vi "Weather Parse Test.vi"() -> ()   [LabVIEW 2020, in "CDM-Config.lvlib"] (continued)
,\n                \"instruction\": null,\n                \"response\": \"Avoid\",\n                \"parameters\": {\n                    \"AWIPSidentifier\": [\n                        \"CWFALU\"\n                    ],\n                    \"WMOidentifier\": [\n                        \"FZAK52 PAFC 031300\"\n                    ],\n                    \"NWSheadline\": [\n                        \"GALE WARNING TODAY\"\n                    ],\n                    \"BLOCKCHANNEL\": [\n                        \"EAS\",\n                        \"NWEM\",\n                        \"CMAS\"\n                    ],\n                    \"VTEC\": [\n                        \"/O.NEW.PAFC.GL.W.5654.251203T1400Z-251204T0200Z/\"\n                    ],\n                    \"eventEndingTime\": [\n                        \"2025-12-03T17:00:00-09:00\"\n                    ]\n                },\n                \"scope\": \"Public\",\n                \"code\": \"IPAWSv1.0\",\n                \"language\": \"en-US\",\n                \"web\": \"http://www.weather.gov\",\n                \"eventCode\": {\n                    \"SAME\": [\n                        \"NWS\"\n                    ],\n                    \"NationalWeatherService\": [\n                        \"GLW\"\n                    ]\n                }\n            }\n        },\n        {\n            \"id\": \"https://api.weather.gov/alerts/urn:oid:2.49.0.1.840.0.16ee1729296b80b5948b72c512c8722f6075ae6c.021.1\",\n            \"type\": \"Feature\",\n            \"geometry\": null,\n            \"properties\": {\n                \"@id\": \"https://api.weather.gov/alerts/urn:oid:2.49.0.1.840.0.16ee1729296b80b5948b72c512c8722f6075ae6c.021.1\",\n                \"@type\": \"wx:Alert\",\n                \"id\": \"urn:oid:2.49.0.1.840.0.16ee1729296b80b5948b72c512c8722f6075ae6c.021.1\",\n                \"areaDesc\": \"Seguam to Adak Bering Side out to 15 NM\",\n                \"geocode\": {\n                    \"SAME\": [\n                        \"058780\"\n                    ],\n                    \"UGC\": [\n                        \"PKZ780\"\n                    ]\n                },\n                \"affectedZones\": [\n                    \"https://api.weather.gov/zones/forecast/PKZ780\"\n                ],\n                \"references\": [],\n                \"sent\": \"2025-12-03T04:00:00-09:00\",\n                \"effective\": \"2025-12-03T04:00:00-09:00\",\n                \"onset\": \"2025-12-03T04:00:00-09:00\",\n                \"expires\": \"2025-12-03T17:00:00-09:00\",\n                \"ends\": \"2025-12-04T05:00:00-09:00\",\n                \"status\": \"Actual\",\n                \"messageType\": \"Alert\",\n                \"category\": \"Met\",\n                \"severity\": \"Moderate\",\n                \"certainty\": \"Likely\",\n                \"urgency\": \"Expected\",\n                \"event\": \"Gale Warning\",\n                \"sender\": \"w-nws.webmaster@noaa.gov\",\n                \"senderName\": \"NWS Anchorage AK\",\n                \"headline\": \"Gale Warning issued December 3 at 4:00AM AKST until December 4 at 5:00AM AKST by NWS Anchorage AK\",\n                \"description\": \"Coastal Waters Forecast for Southwest Alaska+Bristol Bay+The\\nAlaska Peninsula Waters and the Aleutian Islands up to 100 nm out.\\n\\nWind forecasts reflect the predominant speed and direction\\nexpected. Sea forecasts represent an average of the highest\\none-third of the combined wind wave and swell height.\\n\\n.TODAY...N wind 40 kt. Seas 27 ft. Rain.\\n.TONIGHT...N wind 35 kt. Seas 22 ft.\\n.THU...NE wind 25 kt diminishing to 15 kt in the afternoon. Seas\\n16 ft.\\n.THU NIGHT...E wind 15 kt. Seas 10 ft.\\n.FRI...Variable wind 10 kt. Seas 7 ft.\\n.SAT...NE wind 25 kt. Seas 8 ft.\\n.SUN...N wind 30 kt. Seas 20 ft.\",\n                \"instruction\": null,\n                \"response\": \"Avoid\",\n                \"parameters\": {\n                    \"AWIPSidentifier\": [\n                        \"CWFALU\"\n                    ],\n                    \"WMOidentifier\": [\n                        \"FZAK52 PAFC 031300\"\n                    ],\n                    \"NWSheadline\": [\n                        \"GALE WARNING THROUGH TONIGHT\"\n                    ],\n                    \"BLOCKCHANNEL\": [\n                        \"EAS\",\n                        \"NWEM\",\n                        \"CMAS\"\n                    ],\n                    \"VTEC\": [\n                        \"/O.NEW.PAFC.GL.W.5656.251203T1300Z-251204T1400Z/\"\n                    ],\n                    \"eventEndingTime\": [\n                        \"2025-12-04T05:00:00-09:00\"\n                    ]\n                },\n                \"scope\": \"Public\",\n                \"code\": \"IPAWSv1.0\",\n                \"language\": \"en-US\",\n                \"web\": \"http://www.weather.gov\",\n                \"eventCode\": {\n                    \"SAME\": [\n                        \"NWS\"\n                    ],\n                    \"NationalWeatherService\": [\n                        \"GLW\"\n                    ]\n                }\n            }\n        },\n        {\n            \"id\": \"https://api.weather.gov/alerts/urn:oid:2.49.0.1.840.0.16ee1729296b80b5948b72c512c8722f6075ae6c.027.1\",\n            \"type\": \"Feature\",\n            \"geometry\": null,\n            \"properties\": {\n                \"@id\": \"https://api.weather.gov/alerts/urn:oid:2.49.0.1.840.0.16ee1729296b80b5948b72c512c8722f6075ae6c.027.1\",\n                \"@type\": \"wx:Alert\",\n                \"id\": \"urn:oid:2.49.0.1.840.0.16ee1729296b80b5948b72c512c8722f6075ae6c.027.1\",\n                \"areaDesc\": \"Kiska to Attu Bering Side\",\n                \"geocode\": {\n                    \"SAME\": [\n                        \"058786\"\n                    ],\n                    \"UGC\": [\n                        \"PKZ786\"\n                    ]\n                },\n                \"affectedZones\": [\n                    \"https://api.weather.gov/zones/forecast/PKZ786\"\n                ],\n                \"references\": [],\n                \"sent\": \"2025-12-03T04:00:00-09:00\",\n                \"effective\": \"2025-12-03T04:00:00-09:00\",\n                \"onset\": \"2025-12-04T05:00:00-09:00\",\n                \"expires\": \"2025-12-03T17:00:00-09:00\",\n                \"ends\": \"2025-12-04T17:00:00-09:00\",\n                \"status\": \"Actual\",\n                \"messageType\": \"Alert\",\n                \"category\": \"Met\",\n                \"severity\": \"Severe\",\n                \"certainty\": \"Observed\",\n                \"urgency\": \"Immediate\",\n                \"event\": \"Storm Warning\",\n                \"sender\": \"w-nws.webmaster@noaa.gov\",\n                \"senderName\": \"NWS Anchorage AK\",\n                \"headline\": \"Storm Warning issued December 3 at 4:00AM AKST until December 4 at 5:00PM AKST by NWS Anchorage AK\",\n                \"description\": \"Coastal Waters Forecast for Southwest Alaska+Bristol Bay+The\\nAlaska Peninsula Waters and the Aleutian Islands up to 100 nm out.\\n\\nWind forecasts reflect the predominant speed and direction\\nexpected. Sea forecasts represent an average of the highest\\none-third of the combined wind wave and swell height.\\n\\n.TODAY...NE wind 25 kt. Seas 20 ft.\\n.TONIGHT...E wind 30 kt becoming SE 40 kt after midnight. Seas\\n16 ft.\\n.THU...SE wind 50 kt. Seas 19 ft.\\n.THU NIGHT...SE wind 40 kt. Seas 19 ft.\\n.FRI...NW wind 30 kt. Seas 16 ft.\\n.SAT THROUGH SUN...NE wind 20 kt. Seas 12 ft.\",\n                \"instruction\": null,\n                \"response\": \"Avoid\",\n                \"parameters\": {\n                    \"AWIPSidentifier\": [\n                        \"CWFALU\"\n                    ],\n                    \"WMOidentifier\": [\n                        \"FZAK52 PAFC 031300\"\n                    ],\n                    \"NWSheadline\": [\n                        \"STORM WARNING THURSDAY\"\n                    ],\n                    \"BLOCKCHANNEL\": [\n                        \"EAS\",\n                        \"NWEM\",\n                        \"CMAS\"\n                    ],\n                    \"VTEC\": [\n                        \"/O.NEW.PAFC.SR.W.5662.251204T1400Z-251205T0200Z/\"\n                    ],\n                    \"eventEndingTime\": [\n                        \"2025-12-04T17:00:00-09:00\"\n                    ]\n                },\n                \"scope\": \"Public\",\n                \"code\": \"IPAWSv1.0\",\n                \"language\": \"en-US\",\n                \"web\": \"http://www.weather.gov\",\n                \"eventCode\": {\n                    \"SAME\": [\n                        \"NWS\"\n                    ],\n                    \"NationalWeatherService\": [\n                        \"SRW\"\n                    ]\n                }\n            }\n        },\n        {\n            \"id\": \"https://api.weather.gov/alerts/urn:oid:2.49.0.1.840.0.16ee1729296b80b5948b72c512c8722f6075ae6c.012.1\",\n            \"type\": \"Feature\",\n            \"geometry\": null,\n            \"properties\": {\n                \"@id\": \"https://api.weather.gov/alerts/urn:oid:2.49.0.1.840.0.16ee1729296b80b5948b72c512c8722f6075ae6c.012.1\",\n                \"@type\": \"wx:Alert\",\n                \"id\": \"urn:oid:2.49.0.1.840.0.16ee1729296b80b5948b72c512c8722f6075ae6c.012.1\",\n                \"areaDesc\": \"Cape Sarichef to Nikoski Bering Side out to 15 NM\",\n                \"geocode\": {\n                    \"SAME\": [\n                        \"058770\"\n                    ],\n                    \"UGC\": [\n                        \"PKZ770\"\n                    ]\n                },\n                \"affectedZones\": [\n                    \"https://api.weather.gov/zones/forecast/PKZ770\"\n                ],\n                \"references\": [],\n                \"sent\": \"2025-12-03T04:00:00-09:00\",\n                \"effective\": \"2025-12-03T04:00:00-09:00\",\n                \"onset\": \"2025-12-03T04:00:00-09:00\",\n                \"expires\": \"2025-12-03T17:00:00-09:00\",\n                \"ends\": \"2025-12-04T17:00:00-09:00\",\n                \"status\": \"Actual\",\n                \"messageType\": \"Alert\",\n                \"category\": \"Met\",\n                \"severity\": \"Minor\",\n                \"certainty\": \"Likely\",\n                \"urgency\": \"Expected\",\n                \"event\": \"Small Craft Advisory\",\n                \"sender\": \"w-nws.webmaster@noaa.gov\",\n                \"senderName\": \"NWS Anchorage AK\",\n                \"headline\": \"Small Craft Advisory issued December 3 at 4:00AM AKST until December 4 at 5:00PM AKST by NWS Anchorage AK\",\n                \"description\": \"Coastal Waters Forecast for Southwest Alaska+Bristol Bay+The\\nAlaska Peninsula Waters and the Aleutian Islands up to 100 nm out.\\n\\nWind forecasts reflect the predominant speed and direction\\nexpected. Sea forecasts represent an average of the highest\\none-third of the combined wind wave and swell height.\\n\\n.TODAY...NE wind 30 kt. Seas 14 ft. Rain showers.\\n.TONIGHT...N wind 30 kt. Seas 15 ft.\\n.THU...N wind 25 kt. Seas 14 ft.\\n.THU NIGHT...NE wind 20 kt. Seas 10 ft.\\n.FRI...NE wind 25 kt. Seas 7 ft.\\n.SAT...N wind 35 kt. Seas 14 ft.\\n.SUN...N wind 30 kt. Seas 18 ft.\",\n                \"instruction\": null,\n                \"response\": \"Avoid\",\n                \"parameters\": {\n                    \"AWIPSidentifier\": [\n                        \"CWFALU\"\n                    ],\n                    \"WMOidentifier\": [\n                        \"FZAK52 PAFC 031300\"\n                    ],\n                    \"NWSheadline\": [\n                        \"SMALL CRAFT ADVISORY THROUGH THURSDAY\"\n                    ],\n                    \"BLOCKCHANNEL\": [\n                        \"EAS\",\n                        \"NWEM\",\n                        \"CMAS\"\n                    ],\n                    \"VTEC\": [\n                        \"/O.NEW.PAFC.SC.Y.5647.251203T1300Z-251205T0200Z/\"\n                    ],\n                    \"eventEndingTime\": [\n                        \"2025-12-04T17:00:00-09:00\"\n                    ]\n                },\n                \"scope\": \"Public\",\n                \"code\": \"IPAWSv1.0\",\n                \"language\": \"en-US\",\n                \"web\": \"http://www.weather.gov\",\n                \"eventCode\": {\n                    \"SAME\": [\n                        \"NWS\"\n                    ],\n                    \"NationalWeatherService\": [\n                        \"SCY\"\n                    ]\n                }\n            }\n        },\n        {\n            \"id\": \"https://api.weather.gov/alerts/urn:oid:2.49.0.1.840.0.16ee1729296b80b5948b72c512c8722f6075ae6c.009.1\",\n            \"type\": \"Feature\",\n            \"geometry\": null,\n            \"properties\": {\n                \"@id\": \"https://api.weather.gov/alerts/urn:oid:2.49.0.1.840.0.16ee1729296b80b5948b72c512c8722f6075ae6c.009.1\",\n                \"@type\": \"wx:Alert\",\n                \"id\": \"urn:oid:2.49.0.1.840.0.16ee1729296b80b5948b72c512c8722f6075ae6c.009.1\",\n                \"areaDesc\": \"Port Heiden to Nelson Lagoon from 15 to 60 NM\",\n                \"geocode\": {\n                    \"SAME\": [\n                        \"058757\"\n                    ],\n                    \"UGC\": [\n                        \"PKZ757\"\n                    ]\n                },\n                \"affectedZones\": [\n                    \"https://api.weather.gov/zones/forecast/PKZ757\"\n                ],\n                \"references\": [],\n                \"sent\": \"2025-12-03T04:00:00-09:00\",\n                \"effective\": \"2025-12-03T04:00:00-09:00\",\n                \"onset\": \"2025-12-04T05:00:00-09:00\",\n                \"expires\": \"2025-12-03T17:00:00-09:00\",\n                \"ends\": \"2025-12-04T17:00:00-09:00\",\n                \"status\": \"Actual\",\n                \"messageType\": \"Alert\",\n                \"category\": \"Met\",\n                \"severity\": \"Minor\",\n                \"certainty\": \"Likely\",\n                \"urgency\": \"Expected\",\n                \"event\": \"Small Craft Advisory\",\n                \"sender\": \"w-nws.webmaster@noaa.gov\",\n                \"senderName\": \"NWS Anchorage AK\",\n                \"headline\": \"Small Craft Advisory issued December 3 at 4:00AM AKST until December 4 at 5:00PM AKST by NWS Anchorage AK\",\n                \"description\": \"Coastal Waters Forecast for Southwest Alaska+Bristol Bay+The\\nAlaska Peninsula Waters and the Aleutian Islands up to 100 nm out.\\n\\nWind forecasts reflect the predominant speed and direction\\nexpected. Sea forecasts represent an average of the highest\\none-third of the combined wind wave and swell height.\\n\\n.TODAY...E wind 20 kt. Seas 5 ft.\\n.TONIGHT...E wind 20 kt. Seas 6 ft.\\n.THU...NE wind 25 kt. Seas 7 ft.\\n.THU NIGHT...NE wind 25 kt. Seas 7 ft.\\n.FRI...NE wind 35 kt. Seas 11 ft.\\n.SAT...N wind 40 kt. Seas 16 ft.\\n.SUN...NE wind 25 kt. Seas 10 ft.\",\n                \"instruction\": null,\n                \"response\": \"Avoid\",\n                \"parameters\": {\n                    \"AWIPSidentifier\": [\n                        \"CWFALU\"\n                    ],\n                    \"WMOidentifier\": [\n                        \"FZAK52 PAFC 031300\"\n                    ],\n                    \"NWSheadline\": [\n                        \"SMALL CRAFT ADVISORY THURSDAY\"\n                    ],\n                    \"BLOCKCHANNEL\": [\n                        \"EAS\",\n                        \"NWEM\",\n                        \"CMAS\"\n                    ],\n                    \"VTEC\": [\n                        \"/O.NEW.PAFC.SC.Y.5644.251204T1400Z-251205T0200Z/\"\n                    ],\n                    \"eventEndingTime\": [\n                        \"2025-12-04T17:00:00-09:00\"\n                    ]\n                },\n                \"scope\": \"Public\",\n                \"code\": \"IPAWSv1.0\",\n                \"language\": \"en-US\",\n                \"web\": \"http://www.weather.gov\",\n                \"eventCode\": {\n                    \"SAME\": [\n                        \"NWS\"\n                    ],\n                    \"NationalWeatherService\": [\n                        \"SCY\"\n                    ]\n                }\n            }\n        },\n        {\n            \"id\": \"https://api.weather.gov/alerts/urn:oid:2.49.0.1.840.0.16ee1729296b80b5948b72c512c8722f6075ae6c.018.1\",\n            \"type\": \"Feature\",\n            \"geometry\": null,\n            \"properties\": {\n                \"@id\": \"https://api.weather.gov/alerts/urn:oid:2.49.0.1.840.0.16ee1729296b80b5948b72c512c8722f6075ae6c.018.1\",\n                \"@type\": \"wx:Alert\",\n                \"id\": \"urn:oid:2.49.0.1.840.0.16ee1729296b80b5948b72c512c8722f6075ae6c.018.1\",\n                \"areaDesc\": \"Nikolski to Seguam Bering Side from 15 to 85 NM\",\n                \"geocode\": {\n                    \"SAME\": [\n                        \"058776\"\n                    ],\n                    \"UGC\": [\n                        \"PKZ776\"\n                    ]\n                },\n                \"affectedZones\": [\n                    \"https://api.weather.gov/zones/forecast/PKZ776\"\n                ],\n                \"references\": [],\n                \"sent\": \"2025-12-03T04:00:00-09:00\",\n                \"effective\": \"2025-12-03T04:00:00-09:00\",\n                \"onset\": \"2025-12-03T04:00:00-09:00\",\n                \"expires\": \"2025-12-03T17:00:00-09:00\",\n                \"ends\": \"2025-12-04T05:00:00-09:00\",\n                \"status\": \"Actual\",\n                \"messageType\": \"Alert\",\n                \"category\": \"Met\",\n                \"severity\": \"Moderate\",\n                \"certainty\": \"Likely\",\n                \"urgency\": \"Expected\",\n                \"event\": \"Gale Warning\",\n                \"sender\": \"w-nws.webmaster@noaa.gov\",\n                \"senderName\": \"NWS Anchorage AK\",\n                \"headline\": \"Gale Warning issued December 3 at 4:00AM AKST until December 4 at 5:00AM AKST by NWS Anchorage AK\",\n                \"description\": \"Coastal Waters Forecast for Southwest Alaska+Bristol Bay+The\\nAlaska Peninsula Waters and the Aleutian Islands up to 100 nm out.\\n\\nWind forecasts reflect the predominant speed and direction\\nexpected. Sea forecasts represent an average of the highest\\none-third of the combined wind wave and swell height.\\n\\n.TODAY...N wind 35 kt. Seas 25 ft. Rain showers.\\n.TONIGHT...N wind 35 kt. Seas 22 ft.\\n.THU...N wind 30 kt. Seas 16 ft.\\n.THU NIGHT...NE wind 20 kt. Seas 11 ft.\\n.FRI...E wind 15 kt. Seas 8 ft.\\n.SAT...N wind 30 kt. Seas 12 ft.\\n.SUN...N wind 30 kt. Seas 22 ft.\",\n                \"instruction\": null,\n                \"response\": \"Avoid\",\n                \"parameters\": {\n                    \"AWIPSidentifier\": [\n                        \"CWFALU\"\n                    ],\n                    \"WMOidentifier\": [\n                        \"FZAK52 PAFC 031300\"\n                    ],\n                    \"NWSheadline\": [\n                        \"GALE WARNING THROUGH TONIGHT\"\n                    ],\n                    \"BLOCKCHANNEL\": [\n                        \"EAS\",\n                        \"NWEM\",\n                        \"CMAS\"\n                    ],\n                    \"VTEC\": [\n                        \"/O.NEW.PAFC.GL.W.5653.251203T1300Z-251204T1400Z/\"\n                    ],\n                    \"eventEndingTime\": [\n                        \"2025-12-04T05:00:00-09:00\"\n                    ]\n                },\n                \"scope\": \"Public\",\n                \"code\": \"IPAWSv1.0\",\n                \"language\": \"en-US\",\n                \"web\": \"http://www.weather.gov\",\n                \"eventCode\": {\n                    \"SAME\": [\n                        \"NWS\"\n                    ],\n                    \"NationalWeatherService\": [\n                        \"GLW\"\n                    ]\n                }\n            }\n        },\n        {\n            \"id\": \"https://api.weather.gov/alerts/urn:oid:2.49.0.1.840.0.16ee1729296b80b5948b72c512c8722f6075ae6c.024.1\",\n            \"type\": \"Feature\",\n            \"geometry\": null,\n            \"properties\": {\n                \"@id\": \"https://api.weather.gov/alerts/urn:oid:2.49.0.1.840.0.16ee1729296b80b5948b72c512c8722f6075ae6c.024.1\",\n                \"@type\": \"wx:Alert\",\n                \"id\": \"urn:oid:2.49.0.1.840.0.16ee1729296b80b5948b72c512c8722f6075ae6c.024.1\",\n                \"areaDesc\": \"Seguam to Adak Pacific Side from 15 to 75 NM\",\n                \"geocode\": {\n                    \"SAME\": [\n                        \"058783\"\n                    ],\n                    \"UGC\": [\n                        \"PKZ783\"\n                    ]\n                },\n                \"affectedZones\": [\n                    \"https://api.weather.gov/zones/forecast/PKZ783\"\n                ],\n                \"references\": [],\n                \"sent\": \"2025-12-03T04:00:00-09:00\",\n                \"effective\": \"2025-12-03T04:00:00-09:00\",\n                \"onset\": \"2025-12-03T04:00:00-09:00\",\n                \"expires\": \"2025-12-03T17:00:00-09:00\",\n                \"ends\": \"2025-12-04T05:00:00-09:00\",\n                \"status\": \"Actual\",\n                \"messageType\": \"Alert\",\n                \"category\": \"Met\",\n                \"severity\": \"Moderate\",\n                \"certainty\": \"Likely\",\n                \"urgency\": \"Expected\",\n                \"event\": \"Gale Warning\",\n                \"sender\": \"w-nws.webmaster@noaa.gov\",\n                \"senderName\": \"NWS Anchorage AK\",\n                \"headline\": \"Gale Warning issued December 3 at 4:00AM AKST until December 4 at 5:00AM AKST by NWS Anchorage AK\",\n                \"description\": \"Coastal Waters Forecast for Southwest Alaska+Bristol Bay+The\\nAlaska Peninsula Waters and the Aleutian Islands up to 100 nm out.\\n\\nWind forecasts reflect the predominant speed and direction\\nexpected. Sea forecasts represent an average of the highest\\none-third of the combined wind wave and swell height.\\n\\n.TODAY...N wind 40 kt. Seas 17 ft. Rain.\\n.TONIGHT...N wind 35 kt. Seas 15 ft.\\n.THU...N wind 25 kt diminishing to 15 kt in the afternoon. Seas\\n12 ft.\\n.THU NIGHT...NE wind 15 kt. Seas 7 ft.\\n.FRI...S wind 15 kt. Seas 15 ft.\\n.SAT...N wind 25 kt. Seas 11 ft.\\n.SUN...N wind 25 kt. Seas 16 ft.\",\n                \"instruction\": null,\n                \"response\": \"Avoid\",\n                \"parameters\": {\n                    \"AWIPSidentifier\": [\n                        \"CWFALU\"\n                    ],\n                    \"WMOidentifier\": [\n                        \"FZAK52 PAFC 031300\"\n                    ],\n                    \"NWSheadline\": [\n                        \"GALE WARNING THROUGH TONIGHT\"\n                    ],\n                    \"BLOCKCHANNEL\": [\n                        \"EAS\",\n                        \"NWEM\",\n                        \"CMAS\"\n                    ],\n                    \"VTEC\": [\n                        \"/O.NEW.PAFC.GL.W.5659.251203T1300Z-251204T1400Z/\"\n                    ],\n                    \"eventEndingTime\": [\n                        \"2025-12-04T05:00:00-09:00\"\n                    ]\n                },\n                \"scope\": \"Public\",\n                \"code\": \"IPAWSv1.0\",\n                \"language\": \"en-US\",\n                \"web\": \"http://www.weather.gov\",\n                \"eventCode\": {\n                    \"SAME\": [\n                        \"NWS\"\n                    ],\n                    \"NationalWeatherService\": [\n                        \"GLW\"\n                    ]\n                }\n            }\n        },\n        {\n            \"id\": \"https://api.weather.gov/alerts/urn:oid:2.49.0.1.840.0.16ee1729296b80b5948b72c512c8722f6075ae6c.013.1\",\n            \"type\": \"Feature\",\n            \"geometry\": null,\n            \"properties\": {\n                \"@id\": \"https://api.weather.gov/alerts/urn:oid:2.49.0.1.840.0.16ee1729296b80b5948b72c512c8722f6075ae6c.013.1\",\n                \"@type\": \"wx:Alert\",\n                \"id\": \"urn:oid:2.49.0.1.840.0.16ee1729296b80b5948b72c512c8722f6075ae6c.013.1\",\n                \"areaDesc\": \"Cape Sarichef to Nikoski Bering Side from 15 to 85 NM\",\n                \"geocode\": {\n                    \"SAME\": [\n                        \"058772\"\n                    ],\n                    \"UGC\": [\n                        \"PKZ772\"\n                    ]\n                },\n                \"affectedZones\": [\n                    \"https://api.weather.gov/zones/forecast/PKZ772\"\n                ],\n                \"references\": [],\n                \"sent\": \"2025-12-03T04:00:00-09:00\",\n                \"effective\": \"2025-12-03T04:00:00-09:00\",\n                \"onset\": \"2025-12-03T04:00:00-09:00\",\n                \"expires\": \"2025-12-03T17:00:00-09:00\",\n                \"ends\": \"2025-12-04T17:00:00-09:00\",\n                \"status\": \"Actual\",\n                \"messageType\": \"Alert\",\n                \"category\": \"Met\",\n                \"severity\": \"Minor\",\n                \"certainty\": \"Likely\",\n                \"urgency\": \"Expected\",\n                \"event\": \"Small Craft Advisory\",\n                \"sender\": \"w-nws.webmaster@noaa.gov\",\n                \"senderName\": \"NWS Anchorage AK\",\n                \"headline\": \"Small Craft Advisory issued December 3 at 4:00AM AKST until December 4 at 5:00PM AKST by NWS Anchorage AK\",\n                \"description\": \"Coastal Waters Forecast for Southwest Alaska+Bristol Bay+The\\nAlaska Peninsula Waters and the Aleutian Islands up to 100 nm out.\\n\\nWind forecasts reflect the predominant speed and direction\\nexpected. Sea forecasts represent an average of the highest\\none-third of the combined wind wave and swell height.\\n\\n.TODAY...NE wind 30 kt. Seas 16 ft. Rain.\\n.TONIGHT...N wind 30 kt. Seas 17 ft.\\n.THU...N wind 30 kt. Seas 14 ft.\\n.THU NIGHT...NE wind 25 kt. Seas 11 ft.\\n.FRI...NE wind 25 kt. Seas 8 ft.\\n.SAT...N wind 35 kt. Seas 15 ft.\\n.SUN...N wind 35 kt. Seas 21 ft.\",\n                \"instruction\": null,\n                \"response\": \"Avoid\",\n                \"parameters\": {\n                    \"AWIPSidentifier\": [\n                        \"CWFALU\"\n                    ],\n                    \"WMOidentifier\": [\n                        \"FZAK52 PAFC 031300\"\n                    ],\n                    \"NWSheadline\": [\n                        \"SMALL CRAFT ADVISORY THROUGH THURSDAY\"\n                    ],\n                    \"BLOCKCHANNEL\": [\n                        \"EAS\",\n                        \"NWEM\",\n                        \"CMAS\"\n                    ],\n                    \"VTEC\": [\n                        \"/O.NEW.PAFC.SC.Y.5648.251203T1300Z-251205T0200Z/\"\n                    ],\n                    \"eventEndingTime\": [\n                        \"2025-12-04T17:00:00-09:00\"\n                    ]\n                },\n                \"scope\": \"Public\",\n                \"code\": \"IPAWSv1.0\",\n                \"language\": \"en-US\",\n                \"web\": \"http://www.weather.gov\",\n                \"eventCode\": {\n                    \"SAME\": [\n                        \"NWS\"\n                    ],\n                    \"NationalWeatherService\": [\n                        \"SCY\"\n                    ]\n                }\n            }\n        },\n        {\n            \"id\": \"https://api.weather.gov/alerts/urn:oid:2.49.0.1.840.0.16ee1729296b80b5948b72c512c8722f6075ae6c.029.1\",\n            \"type\": \"Feature\",\n            \"geometry\": null,\n            \"properties\": {\n                \"@id\": \"https://api.weather.gov/alerts/urn:oid:2.49.0.1.840.0.16ee1729296b80b5948b72c512c8722f6075ae6c.029.1\",\n                \"@type\": \"wx:Alert\",\n                \"id\": \"urn:oid:2.49.0.1.840.0.16ee1729296b80b5948b72c512c8722f6075ae6c.029.1\",\n                \"areaDesc\": \"Pribilof Islands Nearshore Waters\",\n                \"geocode\": {\n                    \"SAME\": [\n                        \"058766\"\n                    ],\n                    \"UGC\": [\n                        \"PKZ766\"\n                    ]\n                },\n                \"affectedZones\": [\n                    \"https://api.weather.gov/zones/forecast/PKZ766\"\n                ],\n                \"references\": [],\n                \"sent\": \"2025-12-03T04:00:00-09:00\",\n                \"effective\": \"2025-12-03T04:00:00-09:00\",\n                \"onset\": \"2025-12-03T04:00:00-09:00\",\n                \"expires\": \"2025-12-03T17:00:00-09:00\",\n                \"ends\": \"2025-12-04T05:00:00-09:00\",\n                \"status\": \"Actual\",\n                \"messageType\": \"Alert\",\n                \"category\": \"Met\",\n                \"severity\": \"Moderate\",\n                \"certainty\": \"Likely\",\n                \"urgency\": \"Expected\",\n                \"event\": \"Gale Warning\",\n                \"sender\": \"w-nws.webmaster@noaa.gov\",\n                \"senderName\": \"NWS Anchorage AK\",\n                \"headline\": \"Gale Warning issued December 3 at 4:00AM AKST until December 4 at 5:00AM AKST by NWS Anchorage AK\",\n                \"description\": \"Coastal Waters Forecast for Southwest Alaska+Bristol Bay+The\\nAlaska Peninsula Waters and the Aleutian Islands up to 100 nm out.\\n\\nWind forecasts reflect the predominant speed and direction\\nexpected. Sea forecasts represent an average of the highest\\none-third of the combined wind wave and swell height.\\n\\n.TODAY...N wind 40 kt. Seas 19 ft. Rain.\\n.TONIGHT...N wind 35 kt. Seas 16 ft.\\n.THU...NE wind 30 kt. Seas 13 ft.\\n.THU NIGHT...NE wind 25 kt. Seas 10 ft.\\n.FRI...NE wind 25 kt. Seas 8 ft.\\n.SAT...N wind 35 kt. Seas 14 ft.\\n.SUN...N wind 40 kt. Seas 19 ft.\",\n                \"instruction\": null,\n                \"response\": \"Avoid\",\n                \"parameters\": {\n                    \"AWIPSidentifier\": [\n                        \"CWFALU\"\n                    ],\n                    \"WMOidentifier\": [\n                        \"FZAK52 PAFC 031300\"\n                    ],\n                    \"NWSheadline\": [\n                        \"GALE WARNING THROUGH TONIGHT\"\n                    ],\n                    \"BLOCKCHANNEL\": [\n                        \"EAS\",\n                        \"NWEM\",\n                        \"CMAS\"\n                    ],\n                    \"VTEC\": [\n                        \"/O.NEW.PAFC.GL.W.5664.251203T1300Z-251204T1400Z/\"\n                    ],\n                    \"eventEndingTime\": [\n                        \"2025-12-04T05:00:00-09:00\"\n                    ]\n                },\n                \"scope\": \"Public\",\n                \"code\": \"IPAWSv1.0\",\n                \"language\": \"en-US\",\n                \"web\": \"http://www.weather.gov\",\n                \"eventCode\": {\n                    \"SAME\": [\n                        \"NWS\"\n                    ],\n                    \"NationalWeatherService\": [\n                        \"GLW\"\n                    ]\n                }\n            }\n        },\n        {\n            \"id\": \"https://api.weather.gov/alerts/urn:oid:2.49.0.1.840.0.16ee1729296b80b5948b72c512c8722f6075ae6c.026.1\",\n            \"type\": \"Feature\",\n            \"geometry\": null,\n            \"properties\": {\n                \"@id\": \"https://api.weather.gov/alerts/urn:oid:2.49.0.1.840.0.16ee1729296b80b5948b72c512c8722f6075ae6c.026.1\",\n                \"@type\": \"wx:Alert\",\n                \"id\": \"urn:oid:2.49.0.1.840.0.16ee1729296b80b5948b72c512c8722f6075ae6c.026.1\",\n                \"areaDesc\": \"Adak to Kiska Pacific Side\",\n                \"geocode\": {\n                    \"SAME\": [\n                        \"058785\"\n                    ],\n                    \"UGC\": [\n                        \"PKZ785\"\n                    ]\n                },\n                \"affectedZones\": [\n                    \"https://api.weather.gov/zones/forecast/PKZ785\"\n                ],\n                \"references\": [],\n                \"sent\": \"2025-12-03T04:00:00-09:00\",\n                \"effective\": \"2025-12-03T04:00:00-09:00\",\n                \"onset\": \"2025-12-03T05:00:00-09:00\",\n                \"expires\": \"2025-12-03T17:00:00-09:00\",\n                \"ends\": \"2025-12-03T17:00:00-09:00\",\n                \"status\": \"Actual\",\n                \"messageType\": \"Alert\",\n                \"category\": \"Met\",\n                \"severity\": \"Moderate\",\n                \"certainty\": \"Likely\",\n                \"urgency\": \"Expected\",\n                \"event\": \"Gale Warning\",\n                \"sender\": \"w-nws.webmaster@noaa.gov\",\n                \"senderName\": \"NWS Anchorage AK\",\n                \"headline\": \"Gale Warning issued December 3 at 4:00AM AKST until December 3 at 5:00PM AKST by NWS Anchorage AK\",\n                \"description\": \"Coastal Waters Forecast for Southwest Alaska+Bristol Bay+The\\nAlaska Peninsula Waters and the Aleutian Islands up to 100 nm out.\\n\\nWind forecasts reflect the predominant speed and direction\\nexpected. Sea forecasts represent an average of the highest\\none-third of the combined wind wave and swell height.\\n\\n.TODAY...N wind 35 kt. Seas 19 ft.\\n.TONIGHT...N wind 30 kt. Seas 15 ft.\\n.THU...E wind 25 kt. Seas 10 ft.\\n.THU NIGHT...SE wind 30 kt. Seas 11 ft.\\n.FRI...NW wind 30 kt. Seas 16 ft.\\n.SAT...NE wind 20 kt. Seas 11 ft.\\n.SUN...NE wind 25 kt. Seas 12 ft.\",\n                \"instruction\": null,\n                \"response\": \"Avoid\",\n                \"parameters\": {\n                    \"AWIPSidentifier\": [\n                        \"CWFALU\"\n                    ],\n                    \"WMOidentifier\": [\n                        \"FZAK52 PAFC 031300\"\n                    ],\n                    \"NWSheadline\": [\n                        \"GALE WARNING TODAY\"\n                    ],\n                    \"BLOCKCHANNEL\": [\n                        \"EAS\",\n                        \"NWEM\",\n                        \"CMAS\"\n                    ],\n                    \"VTEC\": [\n                        \"/O.NEW.PAFC.GL.W.5661.251203T1400Z-251204T0200Z/\"\n                    ],\n                    \"eventEndingTime\": [\n                        \"2025-12-03T17:00:00-09:00\"\n                    ]\n                },\n                \"scope\": \"Public\",\n                \"code\": \"IPAWSv1.0\",\n                \"language\": \"en-US\",\n                \"web\": \"http://www.weather.gov\",\n                \"eventCode\": {\n                    \"SAME\": [\n                        \"NWS\"\n                    ],\n                    \"NationalWeatherService\": [\n                        \"GLW\"\n                    ]\n                }\n            }\n        },\n        {\n            \"id\": \"https://api.weather.gov/alerts/urn:oid:2.49.0.1.840.0.16ee1729296b80b5948b72c512c8722f6075ae6c.033.2\",\n            \"type\": \"Feature\",\n            \"geometry\": null,\n            \"properties\": {\n                \"@id\": \"https://api.weather.gov/alerts/urn:oid:2.49.0.1.840.0.16ee1729296b80b5948b72c512c8722f6075ae6c.033.2\",\n                \"@type\": \"wx:Alert\",\n                \"id\": \"urn:oid:2.49.0.1.840.0.16ee1729296b80b5948b72c512c8722f6075ae6c.033.2\",\n                \"areaDesc\": \"Kuskokwim Delta and Etolin Strait out to 15 NM\",\n                \"geocode\": {\n                    \"SAME\": [\n                        \"058763\"\n                    ],\n                    \"UGC\": [\n                        \"PKZ763\"\n                    ]\n                },\n                \"affectedZones\": [\n                    \"https://api.weather.gov/zones/forecast/PKZ763\"\n                ],\n                \"references\": [],\n                \"sent\": \"2025-12-03T04:00:00-09:00\",\n                \"effective\": \"2025-12-03T04:00:00-09:00\",\n                \"onset\": \"2025-12-03T04:00:00-09:00\",\n                \"expires\": \"2025-12-03T17:00:00-09:00\",\n                \"ends\": \"2025-12-04T17:00:00-09:00\",\n                \"status\": \"Actual\",\n                \"messageType\": \"Alert\",\n                \"category\": \"Met\",\n                \"severity\": \"Minor\",\n                \"certainty\": \"Likely\",\n                \"urgency\": \"Expected\",\n                \"event\": \"Small Craft Advisory\",\n                \"sender\": \"w-nws.webmaster@noaa.gov\",\n                \"senderName\": \"NWS Anchorage AK\",\n                \"headline\": \"Small Craft Advisory issued December 3 at 4:00AM AKST until December 4 at 5:00PM AKST by NWS Anchorage AK\",\n                \"description\": \"Coastal Waters Forecast for Southwest Alaska+Bristol Bay+The\\nAlaska Peninsula Waters and the Aleutian Islands up to 100 nm out.\\n\\nWind forecasts reflect the predominant speed and direction\\nexpected. Sea forecasts represent an average of the highest\\none-third of the combined wind wave and swell height.\\n\\n.TODAY...NE wind 25 kt. Seas in ice free waters 4 ft. Heavy freezing\\nspray.\\n.TONIGHT...N wind 30 kt. Seas in ice free waters 4 ft. Heavy\\nfreezing spray.\\n.THU...N wind 25 kt. Seas in ice free waters 4 ft. Heavy freezing\\nspray.\\n.THU NIGHT...NE wind 25 kt. Seas in ice free waters 3 ft.\\n.FRI...N wind 40 kt. Seas in ice free waters 5 ft.\\n.SAT...N wind 45 kt. Seas in ice free waters 7 ft.\\n.SUN...N wind 40 kt. Seas in ice free waters 6 ft.\",\n                \"instruction\": null,\n                \"response\": \"Avoid\",\n                \"parameters\": {\n                    \"AWIPSidentifier\": [\n                        \"CWFALU\"\n                    ],\n                    \"WMOidentifier\": [\n                        \"FZAK52 PAFC 031300\"\n                    ],\n                    \"NWSheadline\": [\n                        \"HEAVY FREEZING SPRAY WARNING THROUGH THURSDAY... ...SMALL CRAFT ADVISORY THROUGH THURSDAY\"\n                    ],\n                    \"BLOCKCHANNEL\": [\n                        \"EAS\",\n                        \"NWEM\",\n                        \"CMAS\"\n                    ],\n                    \"VTEC\": [\n                        \"/O.NEW.PAFC.SC.Y.5668.251203T1300Z-251205T0200Z/\"\n                    ],\n                    \"eventEndingTime\": [\n                        \"2025-12-04T17:00:00-09:00\"\n                    ]\n                },\n                \"scope\": \"Public\",\n                \"code\": \"IPAWSv1.0\",\n                \"language\": \"en-US\",\n                \"web\": \"http://www.weather.gov\",\n                \"eventCode\": {\n                    \"SAME\": [\n                        \"NWS\"\n                    ],\n                    \"NationalWeatherService\": [\n                        \"SCY\"\n                    ]\n                }\n            }\n        },\n        {\n            \"id\": \"https://api.weather.gov/alerts/urn:oid:2.49.0.1.840.0.16ee1729296b80b5948b72c512c8722f6075ae6c.020.1\",\n            \"type\": \"Feature\",\n            \"geometry\": null,\n            \"properties\": {\n                \"@id\": \"https://api.weather.gov/alerts/urn:oid:2.49.0.1.840.0.16ee1729296b80b5948b72c512c8722f6075ae6c.020.1\",\n                \"@type\": \"wx:Alert\",\n                \"id\": \"urn:oid:2.49.0.1.840.0.16ee1729296b80b5948b72c512c8722f6075ae6c.020.1\",\n                \"areaDesc\": \"Nikolski to Seguam Pacific Side from 15 to 75 NM\",\n                \"geocode\": {\n                    \"SAME\": [\n                        \"058778\"\n                    ],\n                    \"UGC\": [\n                        \"PKZ778\"\n                    ]\n                },\n                \"affectedZones\": [\n                    \"https://api.weather.gov/zones/forecast/PKZ778\"\n                ],\n                \"references\": [],\n                \"sent\": \"2025-12-03T04:00:00-09:00\",\n                \"effective\": \"2025-12-03T04:00:00-09:00\",\n                \"onset\": \"2025-12-03T04:00:00-09:00\",\n                \"expires\": \"2025-12-03T17:00:00-09:00\",\n                \"ends\": \"2025-12-04T17:00:00-09:00\",\n                \"status\": \"Actual\",\n                \"messageType\": \"Alert\",\n                \"category\": \"Met\",\n                \"severity\": \"Minor\",\n                \"certainty\": \"Likely\",\n                \"urgency\": \"Expected\",\n                \"event\": \"Small Craft Advisory\",\n                \"sender\": \"w-nws.webmaster@noaa.gov\",\n                \"senderName\": \"NWS Anchorage AK\",\n                \"headline\": \"Small Craft Advisory issued December 3 at 4:00AM AKST until December 4 at 5:00PM AKST by NWS Anchorage AK\",\n                \"description\": \"Coastal Waters Forecast for Southwest Alaska+Bristol Bay+The\\nAlaska Peninsula Waters and the Aleutian Islands up to 100 nm out.\\n\\nWind forecasts reflect the predominant speed and direction\\nexpected. Sea forecasts represent an average of the highest\\none-third of the combined wind wave and swell height.\\n\\n.TODAY...N wind 30 kt. Seas 19 ft.\\n.TONIGHT...N wind 30 kt. Seas 19 ft.\\n.THU...N wind 30 kt diminishing to 20 kt in the afternoon. Seas\\n15 ft.\\n.THU NIGHT...N wind 15 kt. Seas 9 ft.\\n.FRI...NE wind 20 kt. Seas 7 ft.\\n.SAT...N wind 25 kt. Seas 10 ft.\\n.SUN...N wind 25 kt. Seas 16 ft.\",\n                \"instruction\": null,\n                \"response\": \"Avoid\",\n                \"parameters\": {\n                    \"AWIPSidentifier\": [\n                        \"CWFALU\"\n                    ],\n                    \"WMOidentifier\": [\n                        \"FZAK52 PAFC 031300\"\n                    ],\n                    \"NWSheadline\": [\n                        \"SMALL CRAFT ADVISORY THROUGH THURSDAY\"\n                    ],\n                    \"BLOCKCHANNEL\": [\n                        \"EAS\",\n                        \"NWEM\",\n                        \"CMAS\"\n                    ],\n                    \"VTEC\": [\n                        \"/O.NEW.PAFC.SC.Y.5655.251203T1300Z-251205T0200Z/\"\n                    ],\n                    \"eventEndingTime\": [\n                        \"2025-12-04T17:00:00-09:00\"\n                    ]\n                },\n                \"scope\": \"Public\",\n                \"code\": \"IPAWSv1.0\",\n                \"language\": \"en-US\",\n                \"web\": \"http://www.weather.gov\",\n                \"eventCode\": {\n                    \"SAME\": [\n                        \"NWS\"\n                    ],\n                    \"NationalWeatherService\": [\n                        \"SCY\"\n                    ]\n                }\n            }\n        },\n        {\n            \"id\": \"https://api.weather.gov/alerts/urn:oid:2.49.0.1.840.0.16ee1729296b80b5948b72c512c8722f6075ae6c.028.1\",\n            \"type\": \"Feature\",\n            \"geometry\": null,\n            \"properties\": {\n                \"@id\": \"https://api.weather.gov/alerts/urn:oid:2.49.0.1.840.0.16ee1729296b80b5948b72c512c8722f6075ae6c.028.1\",\n                \"@type\": \"wx:Alert\",\n                \"id\": \"urn:oid:2.49.0.1.840.0.16ee1729296b80b5948b72c512c8722f6075ae6c.028.1\",\n                \"areaDesc\": \"Kiska to Attu Pacific Side\",\n                \"geocode\": {\n                    \"SAME\": [\n                        \"058787\"\n                    ],\n                    \"UGC\": [\n                        \"PKZ787\"\n                    ]\n                },\n                \"affectedZones\": [\n                    \"https://api.weather.gov/zones/forecast/PKZ787\"\n                ],\n                \"references\": [],\n                \"sent\": \"2025-12-03T04:00:00-09:00\",\n                \"effective\": \"2025-12-03T04:00:00-09:00\",\n                \"onset\": \"2025-12-04T05:00:00-09:00\",\n                \"expires\": \"2025-12-03T17:00:00-09:00\",\n                \"ends\": \"2025-12-04T17:00:00-09:00\",\n                \"status\": \"Actual\",\n                \"messageType\": \"Alert\",\n                \"category\": \"Met\",\n                \"severity\": \"Severe\",\n                \"certainty\": \"Observed\",\n                \"urgency\": \"Immediate\",\n                \"event\": \"Storm Warning\",\n                \"sender\": \"w-nws.webmaster@noaa.gov\",\n                \"senderName\": \"NWS Anchorage AK\",\n                \"headline\": \"Storm Warning issued December 3 at 4:00AM AKST until December 4 at 5:00PM AKST by NWS Anchorage AK\",\n                \"description\": \"Coastal Waters Forecast for Southwest Alaska+Bristol Bay+The\\nAlaska Peninsula Waters and the Aleutian Islands up to 100 nm out.\\n\\nWind forecasts reflect the predominant speed and direction\\nexpected. Sea forecasts represent an average of the highest\\none-third of the combined wind wave and swell height.\\n\\n.TODAY...NE wind 25 kt. Seas 16 ft.\\n.TONIGHT...E wind 35 kt becoming SE 45 kt after midnight. Seas\\n14 ft.\\n.THU...SE wind 50 kt. Seas 22 ft. Rain.\\n.THU NIGHT...S wind 40 kt. Seas 20 ft.\\n.FRI...NW wind 30 kt. Seas 18 ft.\\n.SAT...NE wind 25 kt. Seas 12 ft.\\n.SUN...NE wind 20 kt. Seas 11 ft.\",\n                \"instruction\": null,\n                \"response\": \"Avoid\",\n                \"parameters\": {\n                    \"AWIPSidentifier\": [\n                        \"CWFALU\"\n                    ],\n                    \"WMOidentifier\": [\n                        \"FZAK52 PAFC 031300\"\n                    ],\n                    \"NWSheadline\": [\n                        \"STORM WARNING THURSDAY\"\n                    ],\n                    \"BLOCKCHANNEL\": [\n                        \"EAS\",\n                        \"NWEM\",\n                        \"CMAS\"\n                    ],\n                    \"VTEC\": [\n                        \"/O.NEW.PAFC.SR.W.5663.251204T1400Z-251205T0200Z/\"\n                    ],\n                    \"eventEndingTime\": [\n                        \"2025-12-04T17:00:00-09:00\"\n                    ]\n                },\n                \"scope\": \"Public\",\n                \"code\": \"IPAWSv1.0\",\n                \"language\": \"en-US\",\n                \"web\": \"http://www.weather.gov\",\n                \"eventCode\": {\n                    \"SAME\": [\n                        \"NWS\"\n                    ],\n                    \"NationalWeatherService\": [\n                        \"SRW\"\n                    ]\n                }\n            }\n        },\n        {\n            \"id\": \"https://api.weather.gov/alerts/urn:oid:2.49.0.1.840.0.16ee1729296b80b5948b72c512c8722f6075ae6c.015.1\",\n            \"type\": \"Feature\",\n            \"geometry\": null,\n            \"properties\": {\n                \"@id\": \"https://api.weather.gov/alerts/urn:oid:2.49.0.1.840.0.16ee1729296b80b5948b72c512c8722f6075ae6c.015.1\",\n                \"@type\": \"wx:Alert\",\n                \"id\": \"urn:oid:2.49.0.1.840.0.16ee1729296b80b5948b72c512c8722f6075ae6c.015.1\",\n                \"areaDesc\": \"Cape Sarichef to Nikoski Pacific Side out to 15 NM\",\n                \"geocode\": {\n                    \"SAME\": [\n                        \"058773\"\n                    ],\n                    \"UGC\": [\n                        \"PKZ773\"\n                    ]\n                },\n                \"affectedZones\": [\n                    \"https://api.weather.gov/zones/forecast/PKZ773\"\n                ],\n                \"references\": [],\n                \"sent\": \"2025-12-03T04:00:00-09:00\",\n                \"effective\": \"2025-12-03T04:00:00-09:00\",\n                \"onset\": \"2025-12-03T04:00:00-09:00\",\n                \"expires\": \"2025-12-03T17:00:00-09:00\",\n                \"ends\": \"2025-12-04T17:00:00-09:00\",\n                \"status\": \"Actual\",\n                \"messageType\": \"Alert\",\n                \"category\": \"Met\",\n                \"severity\": \"Minor\",\n                \"certainty\": \"Likely\",\n                \"urgency\": \"Expected\",\n                \"event\": \"Small Craft Advisory\",\n                \"sender\": \"w-nws.webmaster@noaa.gov\",\n                \"senderName\": \"NWS Anchorage AK\",\n                \"headline\": \"Small Craft Advisory issued December 3 at 4:00AM AKST until December 4 at 5:00PM AKST by NWS Anchorage AK\",\n                \"description\": \"Coastal Waters Forecast for Southwest Alaska+Bristol Bay+The\\nAlaska Peninsula Waters and the Aleutian Islands up to 100 nm out.\\n\\nWind forecasts reflect the predominant speed and direction\\nexpected. Sea forecasts represent an average of the highest\\none-third of the combined wind wave and swell height.\\n\\n.TODAY...NE wind 25 kt. Seas 14 ft.\\n.TONIGHT...N wind 25 kt. Seas 9 ft.\\n.THU...N wind 25 kt. Seas 8 ft.\\n.THU NIGHT...NE wind 15 kt. Seas 6 ft.\\n.FRI...NE wind 25 kt. Seas 4 ft.\\n.SAT...N wind 35 kt. Seas 7 ft.\\n.SUN...N wind 30 kt. Seas 7 ft.\",\n                \"instruction\": null,\n                \"response\": \"Avoid\",\n                \"parameters\": {\n                    \"AWIPSidentifier\": [\n                        \"CWFALU\"\n                    ],\n                    \"WMOidentifier\": [\n                        \"FZAK52 PAFC 031300\"\n                    ],\n                    \"NWSheadline\": [\n                        \"SMALL CRAFT ADVISORY THROUGH THURSDAY\"\n                    ],\n                    \"BLOCKCHANNEL\": [\n                        \"EAS\",\n                        \"NWEM\",\n                        \"CMAS\"\n                    ],\n                    \"VTEC\": [\n                        \"/O.NEW.PAFC.SC.Y.5650.251203T1300Z-251205T0200Z/\"\n                    ],\n                    \"eventEndingTime\": [\n                        \"2025-12-04T17:00:00-09:00\"\n                    ]\n                },\n                \"scope\": \"Public\",\n                \"code\": \"IPAWSv1.0\",\n                \"language\": \"en-US\",\n                \"web\": \"http://www.weather.gov\",\n                \"eventCode\": {\n                    \"SAME\": [\n                        \"NWS\"\n                    ],\n                    \"NationalWeatherService\": [\n                        \"SCY\"\n                    ]\n                }\n            }\n        },\n        {\n            \"id\": \"https://api.weather.gov/alerts/urn:oid:2.49.0.1.840.0.16ee1729296b80b5948b72c512c8722f6075ae6c.034.1\",\n            \"type\": \"Feature\",\n            \"geometry\": null,\n            \"properties\": {\n                \"@id\": \"https://api.weather.gov/alerts/urn:oid:2.49.0.1.840.0.16ee1729296b80b5948b72c512c8722f6075ae6c.034.1\",\n                \"@type\": \"wx:Alert\",\n                \"id\": \"urn:oid:2.49.0.1.840.0.16ee1729296b80b5948b72c512c8722f6075ae6c.034.1\",\n                \"areaDesc\": \"Kuskokwim Delta from 15 to 80 NM\",\n                \"geocode\": {\n                    \"SAME\": [\n                        \"058764\"\n                    ],\n                    \"UGC\": [\n                        \"PKZ764\"\n                    ]\n                },\n                \"affectedZones\": [\n                    \"https://api.weather.gov/zones/forecast/PKZ764\"\n                ],\n                \"references\": [],\n                \"sent\": \"2025-12-03T04:00:00-09:00\",\n                \"effective\": \"2025-12-03T04:00:00-09:00\",\n                \"onset\": \"2025-12-03T04:00:00-09:00\",\n                \"expires\": \"2025-12-03T17:00:00-09:00\",\n                \"ends\": \"2025-12-04T17:00:00-09:00\",\n                \"status\": \"Actual\",\n                \"messageType\": \"Alert\",\n                \"category\": \"Met\",\n                \"severity\": \"Minor\",\n                \"certainty\": \"Likely\",\n                \"urgency\": \"Expected\",\n                \"event\": \"Small Craft Advisory\",\n                \"sender\": \"w-nws.webmaster@noaa.gov\",\n                \"senderName\": \"NWS Anchorage AK\",\n                \"headline\": \"Small Craft Advisory issued December 3 at 4:00AM AKST until December 4 at 5:00PM AKST by NWS Anchorage AK\",\n                \"description\": \"Coastal Waters Forecast for Southwest Alaska+Bristol Bay+The\\nAlaska Peninsula Waters and the Aleutian Islands up to 100 nm out.\\n\\nWind forecasts reflect the predominant speed and direction\\nexpected. Sea forecasts represent an average of the highest\\none-third of the combined wind wave and swell height.\\n\\n.TODAY...NE wind 30 kt. Seas 9 ft. Freezing spray.\\n.TONIGHT...NE wind 30 kt. Seas 9 ft. Freezing spray.\\n.THU...NE wind 30 kt. Seas 8 ft. Freezing spray.\\n.THU NIGHT...NE wind 30 kt. Seas 7 ft.\\n.FRI...NE wind 40 kt. Seas 11 ft.\\n.SAT THROUGH SUN...N wind 45 kt. Seas 13 ft.\",\n                \"instruction\": null,\n                \"response\": \"Avoid\",\n                \"parameters\": {\n                    \"AWIPSidentifier\": [\n                        \"CWFALU\"\n                    ],\n                    \"WMOidentifier\": [\n                        \"FZAK52 PAFC 031300\"\n                    ],\n                    \"NWSheadline\": [\n                        \"SMALL CRAFT ADVISORY THROUGH THURSDAY\"\n                    ],\n                    \"BLOCKCHANNEL\": [\n                        \"EAS\",\n                        \"NWEM\",\n                        \"CMAS\"\n                    ],\n                    \"VTEC\": [\n                        \"/O.NEW.PAFC.SC.Y.5669.251203T1300Z-251205T0200Z/\"\n                    ],\n                    \"eventEndingTime\": [\n                        \"2025-12-04T17:00:00-09:00\"\n                    ]\n                },\n                \"scope\": \"Public\",\n                \"code\": \"IPAWSv1.0\",\n                \"language\": \"en-US\",\n                \"web\": \"http://www.weather.gov\",\n                \"eventCode\": {\n                    \"SAME\": [\n                        \"NWS\"\n                    ],\n                    \"NationalWeatherService\": [\n                        \"SCY\"\n                    ]\n                }\n            }\n        },\n        {\n            \"id\": \"https://api.weather.gov/alerts/urn:oid:2.49.0.1.840.0.16ee1729296b80b5948b72c512c8722f6075ae6c.002.1\",\n            \"type\": \"Feature\",\n            \"geometry\": null,\n            \"properties\": {\n                \"@id\": \"https://api.weather.gov/alerts/urn:oid:2.49.0.1.840.0.16ee1729296b80b5948b72c512c8722f6075ae6c.002.1\",\n                \"@type\": \"wx:Alert\",\n                \"id\": \"urn:oid:2.49.0.1.840.0.16ee1729296b80b5948b72c512c8722f6075ae6c.002.1\",\n                \"areaDesc\": \"Sitkinak to Castle Cape out to 15 NM\",\n                \"geocode\": {\n                    \"SAME\": [\n                        \"058750\"\n                    ],\n                    \"UGC\": [\n                        \"PKZ750\"\n                    ]\n                },\n                \"affectedZones\": [\n                    \"https://api.weather.gov/zones/forecast/PKZ750\"\n                ],\n                \"references\": [],\n                \"sent\": \"2025-12-03T04:00:00-09:00\",\n                \"effective\": \"2025-12-03T04:00:00-09:00\",\n                \"onset\": \"2025-12-03T04:00:00-09:00\",\n                \"expires\": \"2025-12-03T17:00:00-09:00\",\n                \"ends\": \"2025-12-04T17:00:00-09:00\",\n                \"status\": \"Actual\",\n                \"messageType\": \"Alert\",\n                \"category\": \"Met\",\n                \"severity\": \"Minor\",\n                \"certainty\": \"Likely\",\n                \"urgency\": \"Expected\",\n                \"event\": \"Small Craft Advisory\",\n                \"sender\": \"w-nws.webmaster@noaa.gov\",\n                \"senderName\": \"NWS Anchorage AK\",\n                \"headline\": \"Small Craft Advisory issued December 3 at 4:00AM AKST until December 4 at 5:00PM AKST by NWS Anchorage AK\",\n                \"description\": \"Coastal Waters Forecast for Southwest Alaska+Bristol Bay+The\\nAlaska Peninsula Waters and the Aleutian Islands up to 100 nm out.\\n\\nWind forecasts reflect the predominant speed and direction\\nexpected. Sea forecasts represent an average of the highest\\none-third of the combined wind wave and swell height.\\n\\n.TODAY...S wind 20 kt. Seas 10 ft.\\n.TONIGHT...SE wind 20 kt. Seas 9 ft. Rain showers.\\n.THU...E wind 20 kt. Seas 9 ft. Rain showers.\\n.THU NIGHT...NE wind 20 kt. Seas 7 ft.\\n.FRI THROUGH SAT...NW wind 35 kt. Seas 7 ft.\\n.SUN...NW wind 25 kt. Seas 5 ft.\",\n                \"instruction\": null,\n                \"response\": \"Avoid\",\n                \"parameters\": {\n                    \"AWIPSidentifier\": [\n                        \"CWFALU\"\n                    ],\n                    \"WMOidentifier\": [\n                        \"FZAK52 PAFC 031300\"\n                    ],\n                    \"NWSheadline\": [\n                        \"SMALL CRAFT ADVISORY THROUGH THURSDAY\"\n                    ],\n                    \"BLOCKCHANNEL\": [\n                        \"EAS\",\n                        \"NWEM\",\n                        \"CMAS\"\n                    ],\n                    \"VTEC\": [\n                        \"/O.NEW.PAFC.SC.Y.5638.251203T1300Z-251205T0200Z/\"\n                    ],\n                    \"eventEndingTime\": [\n                        \"2025-12-04T17:00:00-09:00\"\n                    ]\n                },\n                \"scope\": \"Public\",\n                \"code\": \"IPAWSv1.0\",\n                \"language\": \"en-US\",\n                \"web\": \"http://www.weather.gov\",\n                \"eventCode\": {\n                    \"SAME\": [\n                        \"NWS\"\n                    ],\n                    \"NationalWeatherService\": [\n                        \"SCY\"\n                    ]\n                }\n            }\n        },\n        {\n            \"id\": \"https://api.weather.gov/alerts/urn:oid:2.49.0.1.840.0.16ee1729296b80b5948b72c512c8722f6075ae6c.030.1\",\n            \"type\": \"Feature\",\n            \"geometry\": null,\n            \"properties\": {\n                \"@id\": \"https://api.weather.gov/alerts/urn:oid:2.49.0.1.840.0.16ee1729296b80b5948b72c512c8722f6075ae6c.030.1\",\n                \"@type\": \"wx:Alert\",\n                \"id\": \"urn:oid:2.49.0.1.840.0.16ee1729296b80b5948b72c512c8722f6075ae6c.030.1\",\n                \"areaDesc\": \"Bristol Bay greater than 15 NM\",\n                \"geocode\": {\n                    \"SAME\": [\n                        \"058760\"\n                    ],\n                    \"UGC\": [\n                        \"PKZ760\"\n                    ]\n        
